vi "Copy Columns.vi"(8 "error in (no error)":errorcluster, 10 "Copy Column":refnum<class "Composed Column.lvclass">, 11 "New Column Type":refnum<class "Composed Column.lvclass">) -> (0 "error out":errorcluster, 3 "New Column Out":refnum<class "Composed Column.lvclass">)   [LabVIEW 2020, in "Composed Columns.lvlib" / "Composed Column.lvclass"]
uses:
  Composed Column.lvclass
  Composed Column.lvclass/Composed Column.ctl
  Value Type/Value Type.lvclass
  Check Manager/Constraint Manager.lvclass
  Basic Columns/Column Configuration/Basic Column Configuration Class/Column Configuration.lvclass
  Composed Columns/Value Source Interface Class/Value Source.lvclass
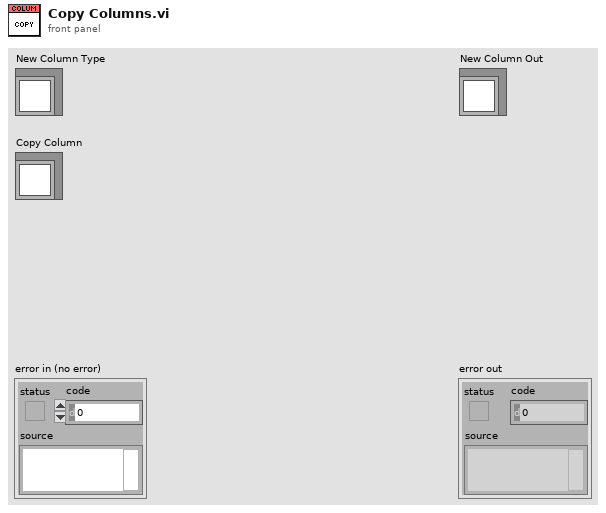
[diagram p1: front panel]
types:
  T1 = cluster{"[0]":refnum<class>, "[1]":refnum<class>, "[2]":refnum<class>, "[3]":refnum<class>}
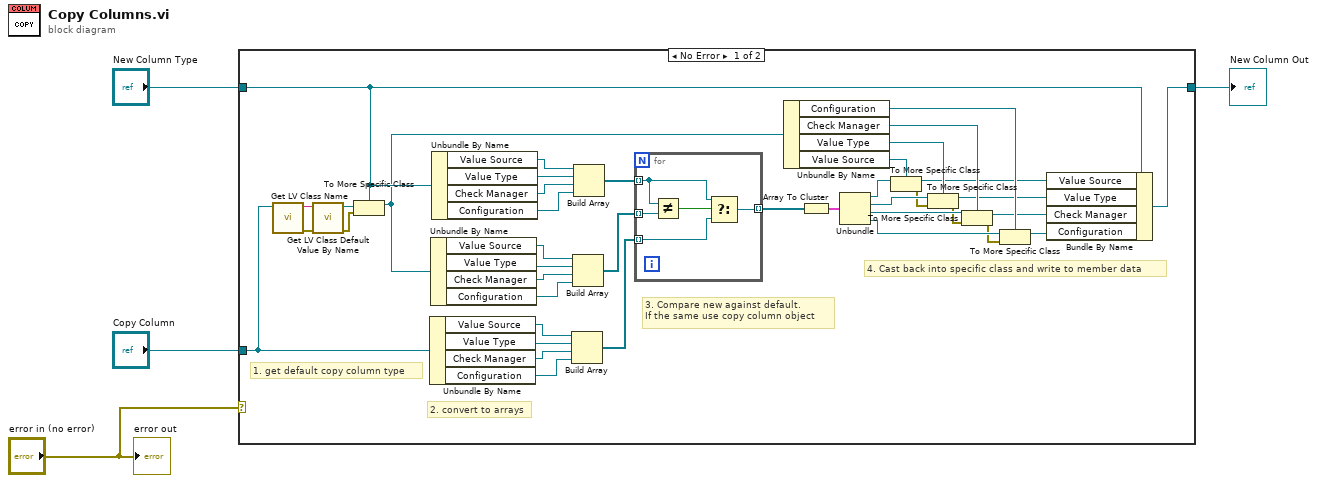
[diagram p0: block diagram]
diagram:
  n1 = case shown="No Error" "error in (no error)" {
    tunnel: "New Column Type" -> [w26 w50]
    tunnel: "Copy Column" -> [w5 _]
    tunnel: [w25 w50] -> w1
    frame No Error {
      # "4. Cast back into specific class and write to member data"
      # "3. Compare new against default.\nIf the same use copy column object"
      # "2. convert to arrays"
      # "1. get default copy column type"
      n2 = call <vilib>:"Get LV Class Name.vi"("object"=w5) -> ("error out"=w44:errorcluster, "class name"=w43:string)  [unwired: 9 in]
      n3 = call <vilib>:"Get LV Class Default Value By Name.vi"("error in (no error)"=w44, "class name"=w43) -> ("error out"=w42:errorcluster, "object"=w41:refnum<class>)  [unwired: 8 in]
      n4 = To More Specific Class(target class=w26, reference=w41, error in=w42) -> (specific class reference=w14:refnum<class "Composed Column.lvclass">)  [unwired: 1 out]
      n5 = Unbundle By Name(w5) -> ("Value Source"=w29:refnum<class "Value Source.lvclass">, "Value Type"=w33:refnum<class "Value Type.lvclass">, "Check Manager"=w32:refnum<class "Constraint Manager.lvclass">, "Configuration"=w31:refnum<class "Column Configuration.lvclass">)
      n6 = Unbundle By Name(w14) -> ("Value Source"=w30:refnum<class "Value Source.lvclass">, "Value Type"=w34:refnum<class "Value Type.lvclass">, "Check Manager"=w35:refnum<class "Constraint Manager.lvclass">, "Configuration"=w36:refnum<class "Column Configuration.lvclass">)
      n7 = Unbundle By Name(w26) -> ("Value Source"=w37:refnum<class "Value Source.lvclass">, "Value Type"=w40:refnum<class "Value Type.lvclass">, "Check Manager"=w39:refnum<class "Constraint Manager.lvclass">, "Configuration"=w38:refnum<class "Column Configuration.lvclass">)
      n8 = Build Array(w29, w33, w32, w31) -> (w27:refnum<class>[])
      n9 = Build Array(w30, w34, w35, w36) -> (w15:refnum<class>[])
      n10 = Build Array(w37, w40, w39, w38) -> (w28:refnum<class>[])
      n11 = for {
        tunnel: w28 -> [w47] mode=indexing
        tunnel: w15 -> [w49] mode=indexing
        tunnel: w27 -> [w46] mode=indexing
        tunnel: [w45] -> w24 mode=indexing
        n12 = Not Equal?(x=w47, y=w49) -> (x != y?=w48:bool)
        n13 = Select(t=w47, s=w48, f=w46) -> (s? t:f=w45:refnum<class>)
      }
      n14 = Unbundle By Name(w14) -> ("Configuration"=w10:refnum<class "Column Configuration.lvclass">, "Check Manager"=w11:refnum<class "Constraint Manager.lvclass">, "Value Type"=w12:refnum<class "Value Type.lvclass">, "Value Source"=w13:refnum<class "Value Source.lvclass">)
      n15 = Array To Cluster(array=w24) -> (cluster=w23:T1)
      n16 = Unbundle(w23) -> ("[0]"=w22:refnum<class>, "[1]"=w21:refnum<class>, "[2]"=w20:refnum<class>, "[3]"=w19:refnum<class>)
      n17 = To More Specific Class(target class=w13, reference=w22) -> (specific class reference=w9:refnum<class "Value Source.lvclass">, error out=w18:errorcluster)  [unwired: 1 in]
      n18 = To More Specific Class(target class=w12, reference=w21, error in=w18) -> (specific class reference=w8:refnum<class "Value Type.lvclass">, error out=w17:errorcluster)
      n19 = To More Specific Class(target class=w11, reference=w20, error in=w17) -> (specific class reference=w7:refnum<class "Constraint Manager.lvclass">, error out=w16:errorcluster)
      n20 = To More Specific Class(target class=w10, reference=w19, error in=w16) -> (specific class reference=w6:refnum<class "Column Configuration.lvclass">)  [unwired: 1 out]
      n21 = Bundle By Name(cluster=w26, "Value Source"=w9, "Value Type"=w8, "Check Manager"=w7, "Configuration"=w6) -> (w25:refnum<class "Composed Column.lvclass">)
    }
    frame Error {
    }
  }
  "New Column Out" <- w1
  "error out" <- "error in (no error)"
